vi "HK Read Value.vi"(8 "error in (no error)":errorcluster, 10 "Channel Name":string, 11 "HK Channel in":refnum<class "HK Table.lvclass">) -> (0 "error out":errorcluster, 1 "Running Avg.":dbl, 2 "Value":dbl, 3 "HK Channel out":refnum<class "HK Table.lvclass">, 4 "Std. Dev.":dbl, 6 "timestamp":timestamp)   [LabVIEW 2024, in "HK Table.lvclass"]
uses:
  HK Table.lvclass
  HK Table.lvclass/HK Table.ctl
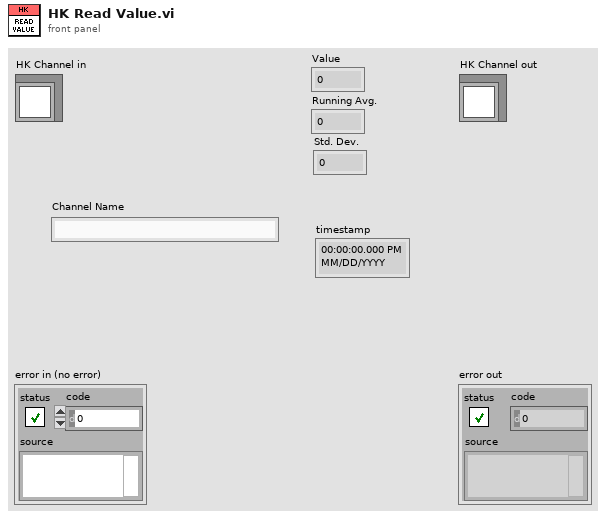
[diagram p1: front panel]
types:
  T1 = typedef "HK Table.lvclass/HK Current Value Table Element.ctl" = cluster{"Value":dbl, "Time Stamp":timestamp, "Running Avg.":dbl, "Std. Dev.":dbl, "Recent Values":dbl[], "Timestamps":timestamp[], "Alarm Status":T2}
  T2 = typedef "HK Item.lvclass/HK Alarm enum Status.ctl" = enum16{"No Alarm", "Red Low", "Red High", "Yellow Low", "Yellow High"}
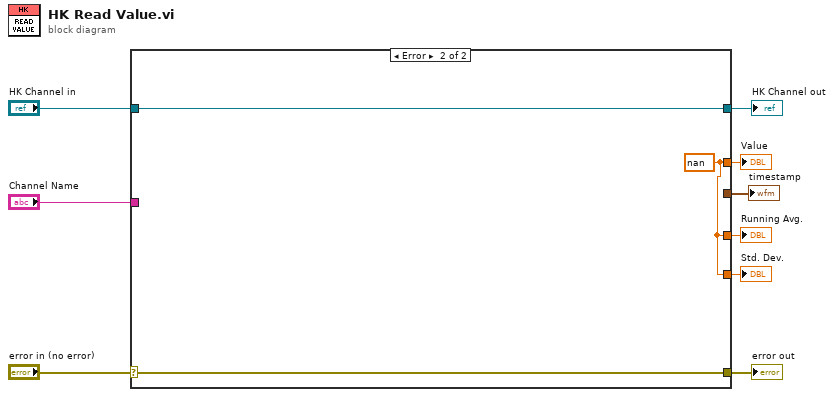
[diagram p0: block diagram]
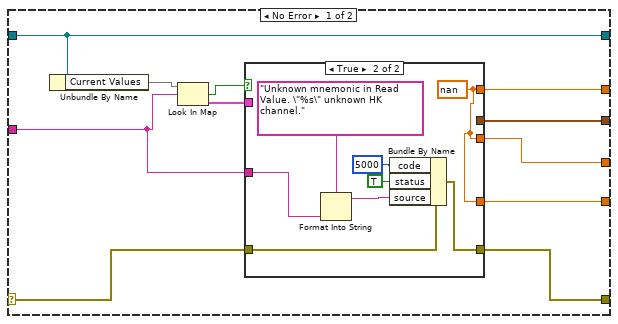
[diagram p2: hidden frame]
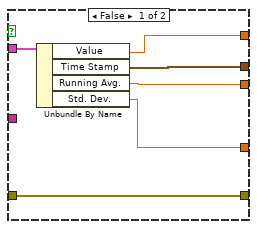
[diagram p3: hidden frame]
diagram:
  n1 = case shown="Error" "error in (no error)" {
    selector: "error in (no error)" -> [w14 w37]
    tunnel: [w13 w37] -> w8
    tunnel: [w20 w36] -> w6
    tunnel: "HK Channel in" -> [w20 w36]
    tunnel: "Channel Name" -> [w12 _]
    tunnel: [w16 w35] -> w4
    tunnel: [w15 w35] -> w2
    tunnel: [w11 _] -> w3
    tunnel: [w10 w35] -> w1
    frame No Error {
      n2 = Unbundle By Name(w20) -> ("Current Values"=w19:map{string, T1})
      n3 = Look In Map(map=w19, key=w12) -> (key not found?=w18:bool, value=w17:T1)  [unwired: 1 in]
      n4 = case shown="True" w18 {
        tunnel: w17 -> [w26 _]
        tunnel: [w25 w27] -> w16
        tunnel: [w24 w27] -> w15
        tunnel: w14 -> [w23 w33]
        tunnel: [w23 w34] -> w13
        tunnel: w12 -> [_ w29]
        tunnel: [w22 _] -> w11
        tunnel: [w21 w27] -> w10
        frame False {
          n5 = Unbundle By Name(w26) -> ("Value"=w25:dbl, "Time Stamp"=w22:timestamp, "Running Avg."=w24:dbl, "Std. Dev."=w21:dbl)
        }
        frame True {
          w27 = nan ("Value")
          n6 = Format Into String(format string="Unknown mnemonic in Read Value. \"%s\" unknown HK channel.", w29) -> (resulting string=w28:string)  [unwired: 2 in, 1 out]
          n7 = Bundle By Name(cluster=w33, "code"=5000, "status"=TRUE, "source"=w28) -> (w34:errorcluster)
        }
      }
    }
    frame Error {
      w35 = nan ("Value")
    }
  }
  "error out" <- w8
  "HK Channel out" <- w6
  "Value" <- w4
  "timestamp" <- w3
  "Running Avg." <- w2
  "Std. Dev." <- w1
